vi "Calculate Button State.vi"(10 "Button State":bool, 11 "Previous Button State":T1=enum."Pressed") -> (3 "New Buton State":T1=enum."Pressed")   [LabVIEW 2021, in "Control State.lvclass"]
uses:
  Control State.lvclass
  Button State.ctl
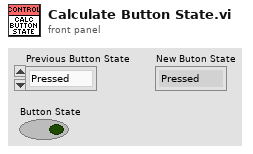
[diagram p1: front panel]
types:
  T1 = typedef "Control State.lvclass/Button State.ctl" = enum16{"Undefined", "Pressed", "Released", "Held", "Not Held"}
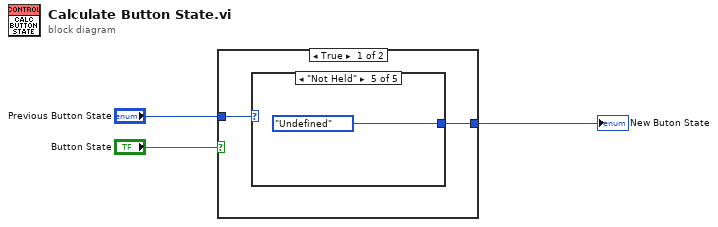
[diagram p0: block diagram]
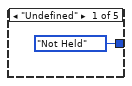
[diagram p2: hidden frame]
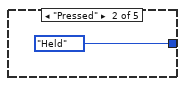
[diagram p3: hidden frame]
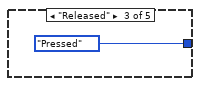
[diagram p4: hidden frame]
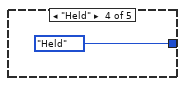
[diagram p5: hidden frame]
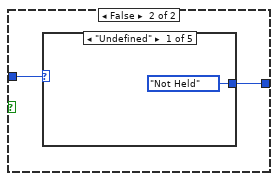
[diagram p6: hidden frame]
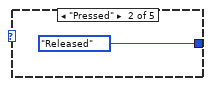
[diagram p7: hidden frame]
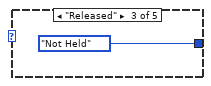
[diagram p8: hidden frame]
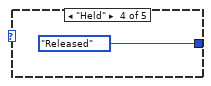
[diagram p9: hidden frame]
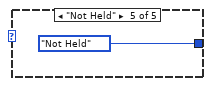
[diagram p10: hidden frame]
diagram:
  n1 = case shown="True" "Button State" {
    tunnel: "Previous Button State" -> [w5 w12]
    tunnel: [w4 w11] -> w3
    frame True {
      n2 = case shown="\"Not Held\"" w5 {
        tunnel: [Button_State."Not Held" ("Primary Weapon") Button_State."Held" ("Primary Weapon") Button_State."Pressed" ("Primary Weapon") Button_State."Held" ("Primary Weapon") Button_State."Undefined" ("Primary Weapon")] -> w4
        frame "Undefined" {
        }
        frame "Pressed" {
        }
        frame "Released" {
        }
        frame "Held" {
        }
        frame "Not Held" {
        }
      }
    }
    frame False {
      n3 = case shown="\"Undefined\"" w12 {
        tunnel: [Button_State."Not Held" ("Primary Weapon") Button_State."Released" ("Primary Weapon") Button_State."Not Held" ("Primary Weapon") Button_State."Released" ("Primary Weapon") Button_State."Not Held" ("Primary Weapon")] -> w11
        frame "Undefined" {
        }
        frame "Pressed" {
        }
        frame "Released" {
        }
        frame "Held" {
        }
        frame "Not Held" {
        }
      }
    }
  }
  "New Buton State" <- w3
